vi "Prepare (pointers).vi"(8 "error in (no error)":errorcluster, 9 "Bytes in SQL":i32, 10 "SQL pointer":i64, 11 "SQLite Connection in":refnum<class "Connection.lvclass">) -> (0 "error out":errorcluster, 1 "Remaining bytes":i32, 2 "Remaining SQL Tail":i64, 3 "SQLite Connection out":refnum<class "Connection.lvclass">, 4 "Valid Statement":bool, 5 "SQL Statement out":refnum<class "SQL Statement.lvclass">)   [LabVIEW 2013, in "SQLiteSupport.lvlib" / "Connection.lvclass"]
doc: "Prepares (compiles) a single SQL statement for later execution. If the SQL contains parameters, then values can be \"bound\" to these parameters using a property node and the \"Bind\" properties. Prepares SQL statements are exectuted by calling \"First Step\". If data is returned it can be accessed using the \"Column\" properties, and multiple returned rows can be stepped through using \"Step\". After completion, the prepared statement can be \"Reset\" and reused, or it can be released (destroyed) using \"Finalize\"."
uses:
  Connection.lvclass
  SQL Statement/SQL Statement.lvclass
  Connection.lvclass/Connection.ctl
  SQL Statement/SQL Statement.lvclass/SQL Statement.ctl
  SQLiteSupport.lvlib
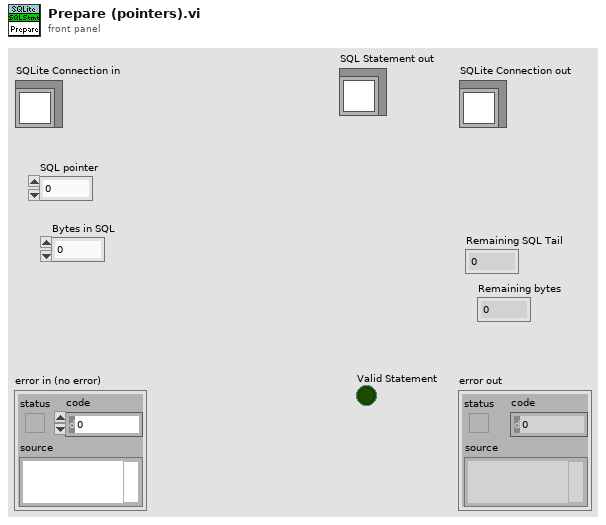
[diagram p1: front panel]
types:
  T1 = typedef "SQLiteSupport.lvlib/SQL Statement.lvclass/Text Encoding" = enum16{"System", "UTF-8", "UTF-16"}
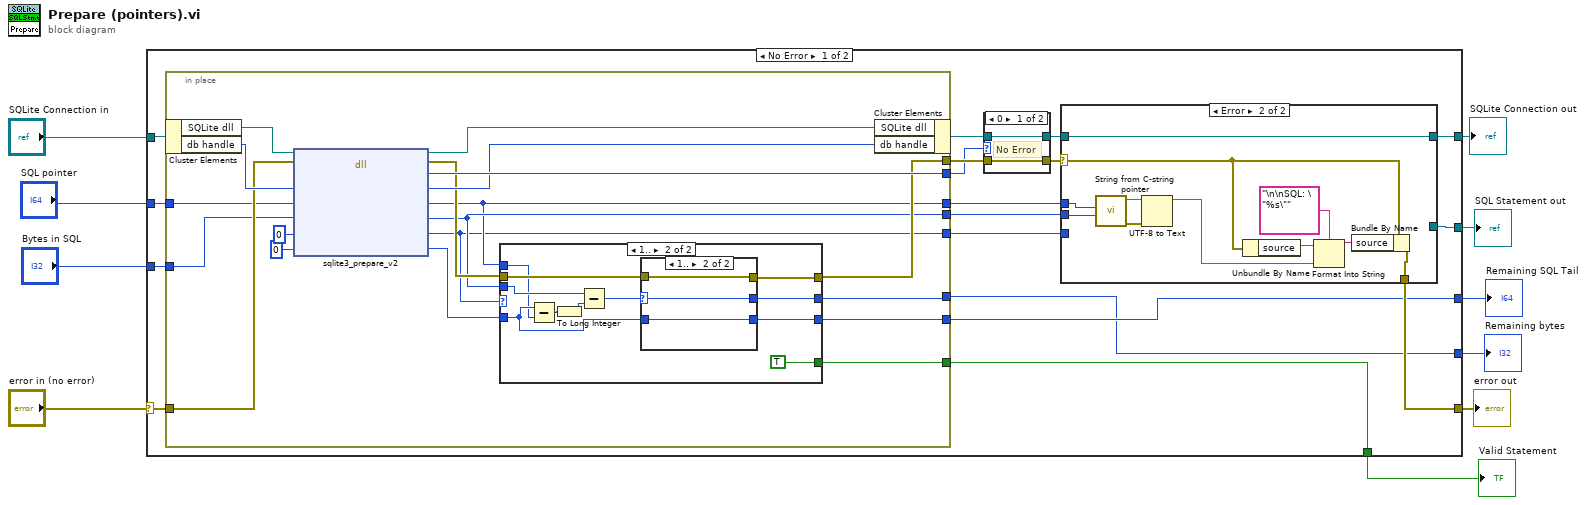
[diagram p0: block diagram]
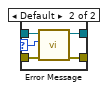
[diagram p4: hidden frame]
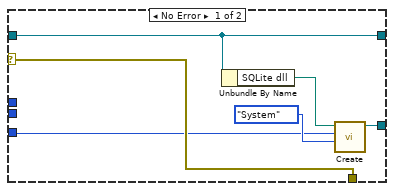
[diagram p5: hidden frame]
diagram:
  n1 = case shown="No Error" "error in (no error)" {
    selector: "error in (no error)" -> [w28 w91]
    tunnel: [w25 w91] -> w9
    tunnel: [w18 w90] -> w7
    tunnel: "SQLite Connection in" -> [w21 w90]
    tunnel: [w26 _] -> w6
    tunnel: [w17 _] -> w5
    tunnel: "SQL pointer" -> [w16 _]
    tunnel: "Bytes in SQL" -> [w15 _]
    tunnel: [w14 _] -> w2
    tunnel: [w13 _] -> w1
    frame No Error {
      n2 = in-place {
        in-place-border: w28 -> [w36]
        in-place-border: [w30] -> w27
        in-place-border: [w37] -> w24
        in-place-border: [w47] -> w22
        in-place-border: [w38] -> w17
        in-place-border: w16 -> [w35]
        in-place-border: w15 -> [w34]
        in-place-border: [w33] -> w13
        in-place-border: [w32] -> w14
        in-place-border: [w31] -> w12
        in-place-border: [w29] -> w11
        n3 = in-place-cluster #1(w21) -> ("SQLite dll"=w46:path, "db handle"=w45:u64)
        n4 = dll-call lib="C:/LabVIEW_JDP/Support/SQLite/SQL Connection/sqlite3.dll" fn="sqlite3_prepare_v2"(path in=w46, error in=w36, "db handle"=w45, "SQL pointer"=w35, "nByte"=w34, "Statement"=u64 0, "Remaining SQL Tail"=i64 0 ("Tail")) -> (path out=w43:path, error out=w39:errorcluster, "return code"=w47:i32, "db handle"=w44:u64, "SQL pointer"=w30:i64, "nByte"=w31:i32, "Statement"=w29:u64, "Remaining SQL Tail"=w40:i64)  [unwired: 1 in]
        n5 = case shown="1.." w29 {
          tunnel: w40 -> [w48 w55]
          tunnel: w39 -> [w49 w60]
          tunnel: [_ TRUE] -> w38
          tunnel: w31 -> [_ w59]
          tunnel: w30 -> [_ w54]
          tunnel: [w49 w56] -> w37
          tunnel: [_ w51] -> w33
          tunnel: [w48 w50] -> w32
          frame ..0 {
            # "Not a valid\nSQL statement"
          }
          frame 1.. {
            n6 = Subtract(x=w55, y=w54) -> (x-y=w58:i64)
            n7 = To Long Integer(number=w58) -> (32bit integer=w57:i32)
            n8 = Subtract(x=w59, y=w57) -> (x-y=w53:i32)
            n9 = case shown="1.." w53 {
              selector: w53 -> [_ w65]
              tunnel: w60 -> [w62 w63]
              tunnel: [w62 w63] -> w56
              tunnel: w55 -> [w61 w64]
              tunnel: [_ w65] -> w51
              tunnel: [w61 w64] -> w50
              frame ..0 {
              }
              frame 1.. {
              }
            }
          }
        }
        n10 = in-place-cluster #1("SQLite dll"=w43, "db handle"=w44) -> (w20:refnum<class "Connection.lvclass">)
      }
      n11 = case shown="0" w22 {
        selector: w22 -> [_ w68]
        tunnel: w20 -> [w67 w72]
        tunnel: [w67 w71] -> w19
        tunnel: w24 -> [w66 w70]
        tunnel: [w66 w69] -> w23
        frame 0 {
          # "No Error"
        }
        frame Default {
          n12 = call "Error Message.vi"("error in (no error)"=w70, "error code"=w68, "Connection in"=w72) -> ("error out"=w69:errorcluster, "Connection out"=w71:refnum<class "Connection.lvclass">)  [unwired: 7 in]
        }
      }
      n13 = case shown="Error" w23 {
        selector: w23 -> [w77 w88]
        tunnel: w27 -> [_ w82]
        tunnel: [w78 _] -> w26
        tunnel: [w77 w89] -> w25
        tunnel: w19 -> [w76 w84]
        tunnel: [w76 w84] -> w18
        tunnel: w12 -> [_ w81]
        tunnel: w11 -> [w73 _]
        frame No Error {
          n14 = Unbundle By Name(w76) -> ("SQLite dll"=w75:path)
          n15 = call "Create.vi"("Encoding"=Text_Encoding."System", "Statement handle"=w73, "SQLite dll"=w75) -> ("SQL Statement out"=w78:refnum<class "SQL Statement.lvclass">)  [unwired: 8 in]
        }
        frame Error {
          n16 = call "String from C-string pointer.vi"("Bytes to copy"=w81, "Pointer"=w82) -> ("error out"=w83:errorcluster, "string"=w80:string)  [unwired: 8 in]
          n17 = UTF-8 to Text(8:w83, 11:w80) -> (3:w79:string)  [unwired: 1 out]
          n18 = Unbundle By Name(w88) -> ("source"=w87:string)
          n19 = Format Into String(format string="\n\nSQL: \"%s\"", initial string=w87, w79) -> (resulting string=w85:string)  [unwired: 1 in, 1 out]
          n20 = Bundle By Name(cluster=w88, "source"=w85) -> (w89:errorcluster)
        }
      }
    }
    frame Error {
    }
  }
  "error out" <- w9
  "SQLite Connection out" <- w7
  "SQL Statement out" <- w6
  "Valid Statement" <- w5
  "Remaining SQL Tail" <- w2
  "Remaining bytes" <- w1
